vi "pos-to-DL.vi"(2 "DL param":cluster{"min":dbl, "max":dbl, "real pos":dbl}, 3 "pos, mm":dbl) -> (0 "pos, mm":dbl, 1 "DL pos":dbl)   [LabVIEW 2019, in "ControlDL.xctl"]
uses:
  ControlDL.xctl
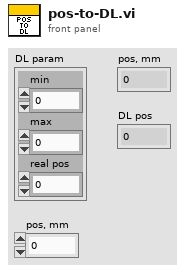
[diagram p1: front panel]
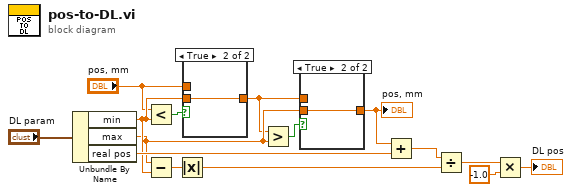
[diagram p0: block diagram]
diagram:
  n1 = Unbundle By Name("DL param") -> ("min"=w10:dbl, "max"=w9:dbl, "real pos"=w13:dbl)
  n2 = Less?(x="pos, mm", y=w10) -> (x < y?=w5:bool)
  n3 = Subtract(x=w9, y=w10) -> (x-y=w11:dbl)
  n4 = Absolute Value(x=w11) -> (abs(x)=w15:dbl)
  n5 = case shown="True" w5 {
    tunnel: w10 -> [_ w17]
    tunnel: [w16 w17] -> w8
    tunnel: "pos, mm" -> [w16 _]
    frame False {
    }
    frame True {
    }
  }
  n6 = Greater?(x=w8, y=w9) -> (0:w6:bool)
  n7 = case shown="True" w6 {
    tunnel: w9 -> [_ w19]
    tunnel: w8 -> [w18 _]
    tunnel: [w18 w19] -> w12
    frame False {
    }
    frame True {
    }
  }
  "pos, mm" <- w12
  n8 = Add(x=w12, y=w13) -> (x+y=w14:dbl)
  n9 = Divide(x=w14, y=w15) -> (x/y=w3:dbl)
  n10 = Multiply(x=w3, y=-1.0) -> (x*y=→"DL pos":dbl)
